vi "Ethernet DIO test.vi"() -> ()   [LabVIEW 2021]
uses:
  Ethernet/Ethernet.lvclass
panel:
  in  "DIO Enable":bool[](array[boolean])
  in  "DIO Direction":bool[](array[boolean])
  out "DIO Readback":bool[](array[boolean])
  in  "UDP port":u16=54321
  in  "TCP port":u16=12345
  in  "Box IP address":string="192.168.1.100"
  out "error out":errorcluster
  in  "stop":bool
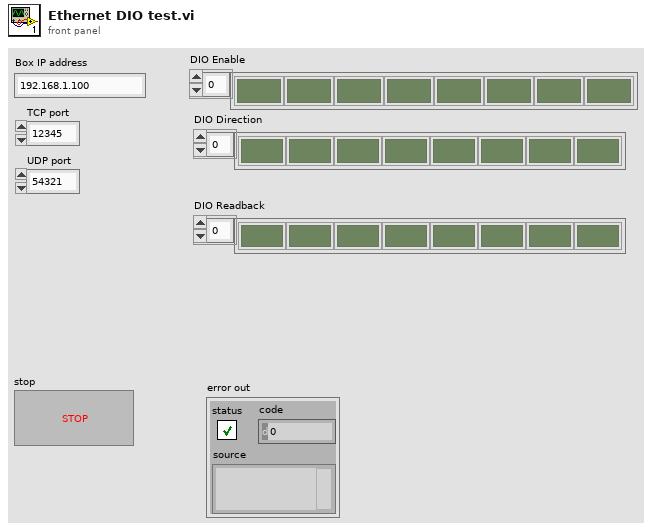
[diagram p1: front panel]
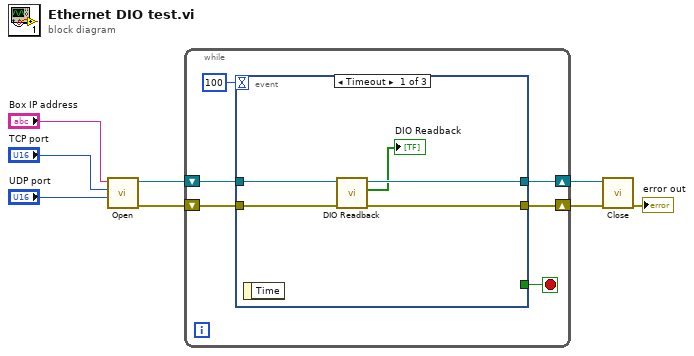
[diagram p0: block diagram]
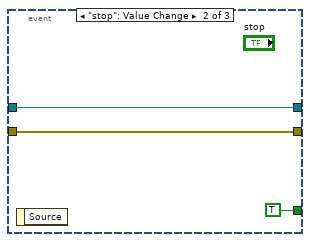
[diagram p2: hidden frame]
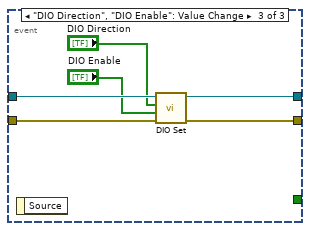
[diagram p3: hidden frame]
diagram:
  n1 = call "Open.vi"("UDP port"="UDP port", "TCP port"="TCP port", "Box IP address"="Box IP address") -> ("error out"=w8:errorcluster, "ENET out"=w7:refnum<class "Ethernet.lvclass">)  [unwired: 7 in]
  n2 = while {
    shift-right: [w11] -> w6
    shift-left: w7 -> [w13]
    shift-right: [w10] -> w5
    shift-left: w8 -> [w12]
    stop <- w9 stop-if-true
    n3 = event shown="[0] Timeout" {
      selector: _ -> [_ _ _]
      dyn-events: _ -> [_ _ _]
      timeout: 100 -> [_ _ _]
      tunnel: w13 -> [w18 w22 w27]
      tunnel: w12 -> [w19 w21 w28]
      tunnel: [w16 w22 w25] -> w11
      tunnel: [w17 w21 w26] -> w10
      tunnel: [_ TRUE _] -> w9
      event Timeout {
        n4 = event-data() -> ()  [unwired: 1 in, 1 out]
        n5 = call-dynamic "DIO Readback.vi"("error in (no error)"=w19, "ENET in"=w18) -> ("error out"=w17:errorcluster, "DIO Readback"=→"DIO Readback":bool[], "ENET out"=w16:refnum<class "Ethernet.lvclass">)  [unwired: 7 in]
      }
      event "stop": Value Change {
        n6 = event-data() -> ()  [unwired: 1 in, 1 out]
      }
      event "DIO Direction", "DIO Enable": Value Change {
        n7 = event-data() -> ()  [unwired: 1 in, 1 out]
        n8 = call-dynamic "DIO Set.vi"("error in (no error)"=w28, "DIO Enable"="DIO Enable", "DIO Direction"="DIO Direction", "ENET in"=w27) -> ("error out"=w26:errorcluster, "ENET out"=w25:refnum<class "Ethernet.lvclass">)  [unwired: 6 in]
      }
    }
  }
  n9 = call-dynamic "Close.vi"("error in (no error)"=w5, "ENET in"=w6) -> ("error out"=→"error out":errorcluster)  [unwired: 9 in]
